vi "Write CAN FIFO.vi"(6 "FIFO Timestamps":T1, 7 "Channel Index":i32, 8 "error in (no error)":errorcluster, 9 "Timeout (ms)":i32, 10 "Data":u8[](array[numeric]) format="%.0x", 11 "CIFCorePlugin in":refnum<class "CIFCorePlugin.lvclass">) -> (0 "error out":errorcluster, 1 "timed out?":bool, 3 "CIFCorePlugin out":refnum<class "CIFCorePlugin.lvclass">)   [LabVIEW 2021, in "CIFCorePlugin.lvclass"]
uses:
  CIFCorePlugin.lvclass
  <vilib>/CIF Foundation/CIF Channels Core/CIFChannels/CIFChannels.lvclass
  <vilib>/CIF Foundation/CIF Channels Core/ChannelCommon/typedef/TimeStamps.ctl
  <vilib>/CIF Foundation/CIF Channels Core/ChannelCommon/ChannelCommon.lvlib
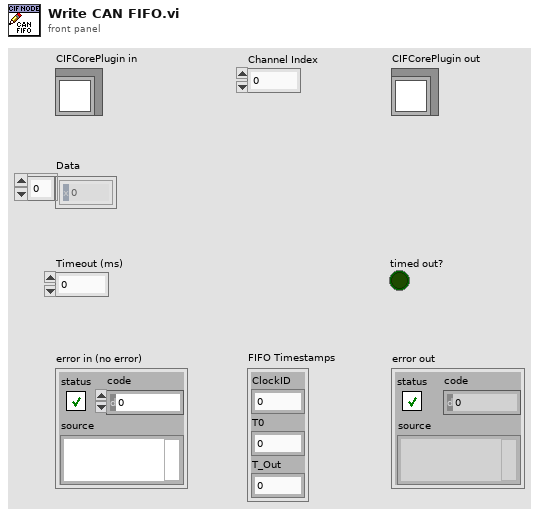
[diagram p1: front panel]
types:
  T1 = typedef "ChannelCommon.lvlib/TimeStamps.ctl" = cluster{"ClockID":u8, "T0":i64, "T_Out":i64}
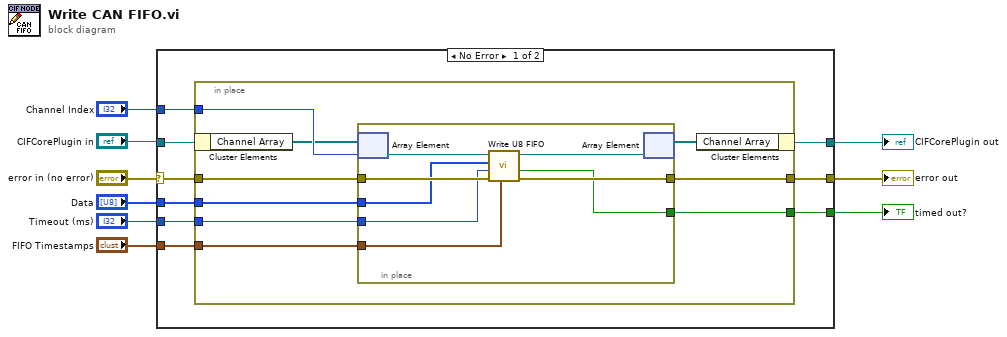
[diagram p0: block diagram]
diagram:
  n1 = case shown="No Error" "error in (no error)" {
    selector: "error in (no error)" -> [w18 w37]
    tunnel: [w17 w37] -> w7
    tunnel: [w15 w36] -> w8
    tunnel: "CIFCorePlugin in" -> [w16 w36]
    tunnel: "Channel Index" -> [w14 _]
    tunnel: "Data" -> [w13 _]
    tunnel: "Timeout (ms)" -> [w12 _]
    tunnel: [w11 _] -> w3
    tunnel: "FIFO Timestamps" -> [w10 _]
    frame No Error {
      n2 = in-place {
        in-place-border: w18 -> [w21]
        in-place-border: [w20] -> w17
        in-place-border: w14 -> [w27]
        in-place-border: w13 -> [w26]
        in-place-border: w12 -> [w25]
        in-place-border: [w24] -> w11
        in-place-border: w10 -> [w23]
        n3 = in-place-cluster #1(w16) -> ("Channel Array"=w22:refnum<class "CIFChannels.lvclass">[])
        n4 = in-place {
          in-place-border: w21 -> [w34]
          in-place-border: [w33] -> w20
          in-place-border: w26 -> [w31]
          in-place-border: w25 -> [w30]
          in-place-border: [w29] -> w24
          in-place-border: w23 -> [w28]
          n5 = in-place-array #2(w22, w27) -> (w35:refnum<class "CIFChannels.lvclass">)
          n6 = call-dynamic "Write U8 FIFO.vi"("FIFO Timestamps"=w28, "error in (no error)"=w34, "Timeout (ms)"=w30, "Data in"=w31, "CIFChannels in"=w35) -> ("error out"=w33:errorcluster, "timed out?"=w29:bool, "CIFChannels out"=w32:refnum<class "CIFChannels.lvclass">)  [unwired: 3 in, 1 out]
          n7 = in-place-array #2(w32) -> (w19:refnum<class "CIFChannels.lvclass">[])  [unwired: 1 out]
        }
        n8 = in-place-cluster #1("Channel Array"=w19) -> (w15:refnum<class "CIFCorePlugin.lvclass">)
      }
    }
    frame Error {
    }
  }
  "error out" <- w7
  "CIFCorePlugin out" <- w8
  "timed out?" <- w3
